vi "DrawlingFigure.vi"() -> ()   [LabVIEW 2015]
uses:
  <vilib>/picture/3D Picture Control/Object/Create Object (name).vi
  <vilib>/picture/3D Picture Control/NI_3D Picture Control.lvlib
panel:
  in  "Scale":cluster{"X":sgl, "Y":sgl, "Z":sgl}
  in  "Axis":cluster{"X":sgl, "Y":sgl, "Z":sgl}
  in  "Angle":sgl
  in  "stop":bool
  out "3D Picture":refnum<vi>(3d-picture)
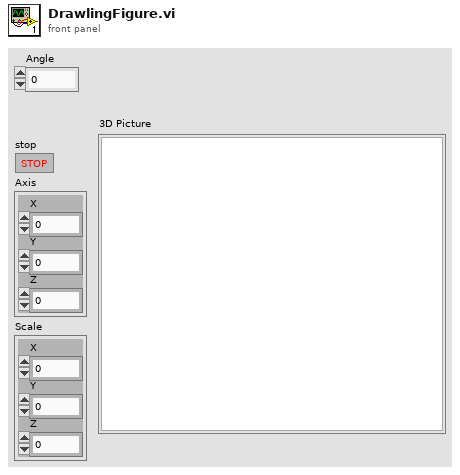
[diagram p1: front panel]
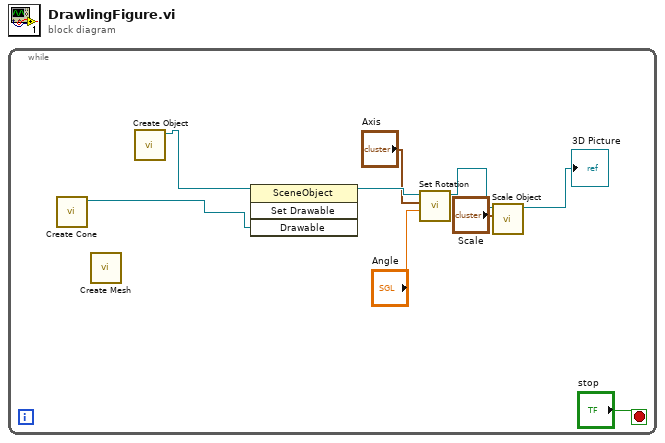
[diagram p0: block diagram]
diagram:
  n1 = while {
    stop <- "stop" stop-if-true
    n2 = call <vilib>:"Create Cone.vi"() -> ("New Cone Refnum"=w7:refnum<vi>)  [unwired: 10 in, 1 out]
    n3 = call <vilib>:"Create Mesh.vi"() -> ()  [unwired: 10 in, 2 out]
    n4 = call-poly <vilib>:"Create Object.vi"() -> ("Scene:New Object"=w9:refnum<vi>)  [unwired: 10 in, 1 out]
    n5 = invoke class="SceneObject" method="Set Drawable"(reference=w9, "Drawable"=w7) -> (reference out=w6:refnum<vi>)  [unwired: 2 in, 3 out]
    n6 = call <vilib>:"Set Rotation.vi"("Angle"="Angle", "Axis"="Axis", "Scene Object"=w6) -> ("Rotated Scene Object"=w3:refnum<vi>)  [unwired: 7 in, 1 out]
    n7 = call <vilib>:"Scale Object.vi"("Scale"="Scale", "Scene.Object In"=w3) -> ("Scene.Object Out"=→"3D Picture":refnum<vi>)  [unwired: 8 in, 1 out]
  }
